vi "Write Element of EIS_ResultsV2.vi"(8 "error in (no error)":errorcluster, 9 "Numeric":dbl, 10 "indices":i32[](array[numeric]), 11 "ChirpV2 in":refnum<class "ChirpV2.lvclass">) -> (0 "error out":errorcluster, 3 "ChirpV2 out":refnum<class "ChirpV2.lvclass">)   [LabVIEW 2014, in "ChirpV2.lvclass"]
uses:
  ChirpV2.lvclass
  ChirpV2.lvclass/ChirpV2.ctl
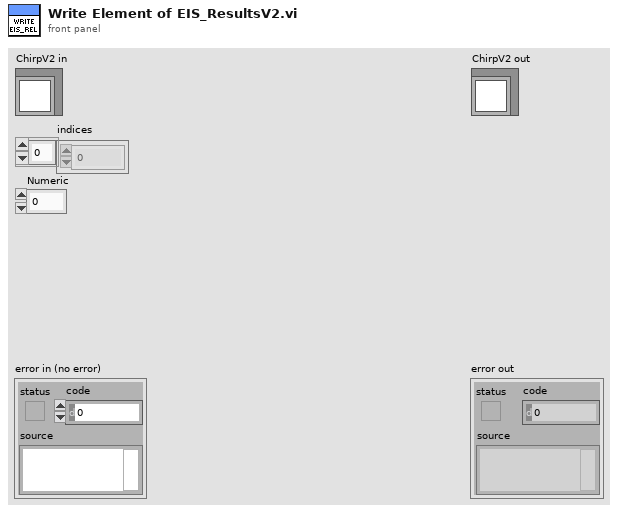
[diagram p1: front panel]
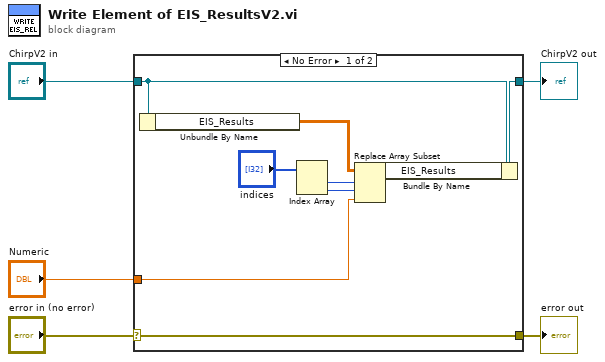
[diagram p0: block diagram]
diagram:
  n1 = case shown="No Error" "error in (no error)" {
    selector: "error in (no error)" -> [w14 w15]
    tunnel: [w14 w15] -> w4
    tunnel: [w13 w16] -> w2
    tunnel: "ChirpV2 in" -> [w6 w16]
    tunnel: "Numeric" -> [w7 _]
    frame No Error {
      n2 = Unbundle By Name(w6) -> ("EIS_Results"=w8:dbl[][])
      n3 = Index Array(array="indices") -> (element #1=w10:i32, element #2=w9:i32)  [unwired: 2 in]
      n4 = Replace Array Subset(array=w8, new element=w7, index (row)=w10, index (col)=w9) -> (w12:dbl[][])
      n5 = Bundle By Name(cluster=w6, "EIS_Results"=w12) -> (w13:refnum<class "ChirpV2.lvclass">)
    }
    frame Error {
    }
  }
  "error out" <- w4
  "ChirpV2 out" <- w2
